vi "System Set Points and States.vi"() -> ()   [LabVIEW 2011]
panel:
  out "Left Encoder SetPoint":dbl
  out "Right Encoder SetPoint":dbl
  in  "Track Target":bool
  out "Indexer Dist":dbl
  out "Shooter RPM":dbl
  out "Indexer RPM":dbl
  out "Open Loop PWM":dbl
  in  "Open Loop":bool
  in  "Shooter Enabled":bool
  out "Hood Voltage":dbl
  out "ShooterSet Speed":dbl
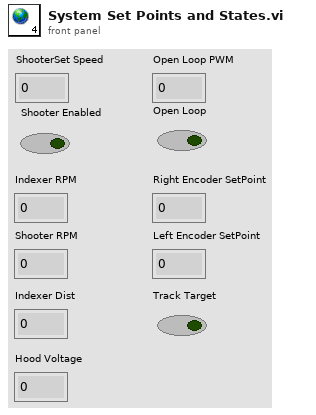
[diagram p1: front panel]
diagram:
